vi "meTEC_Read_ID 101_Hardware Version.vi"(8 "error in (no error)":errorcluster, 9 "TEC Configuration_IN":T1={"VISA resource name"="", "Device Address"=2}, 10 "Sequence No.":u32=5552) -> (0 "error out":errorcluster, 1 "TEC Configuration_OUT":T1={"VISA resource name"="", "Device Address"=2}, 2 "Hardware Version (ID 101) [I32]":i32, 3 "Hardware Version (ID 101) [String]":string)   [LabVIEW 2023]
uses:
  TypeDefs/meTEC_Configuration.ctl
panel:
  # "--- Inputs ---"
  # "--- Outputs ---"
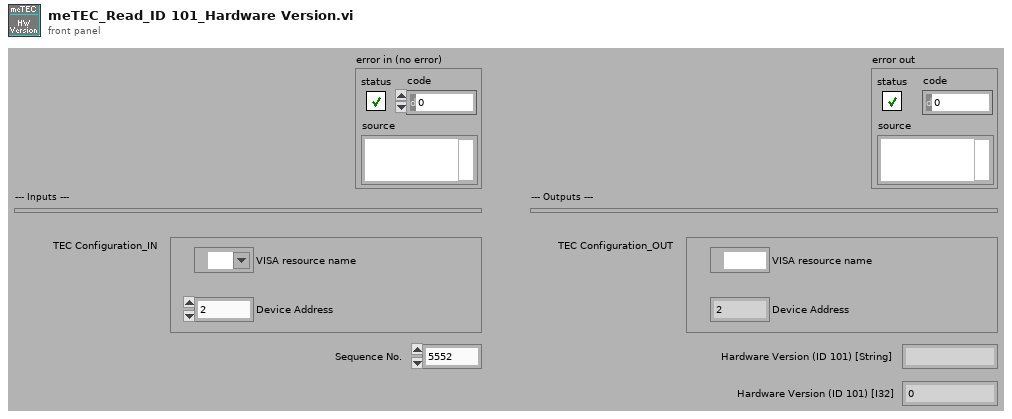
[diagram p1: front panel]
types:
  T1 = typedef "meTEC_Configuration.ctl" = cluster{"VISA resource name":refnum<visa-resource-name>, "Device Address":u16}
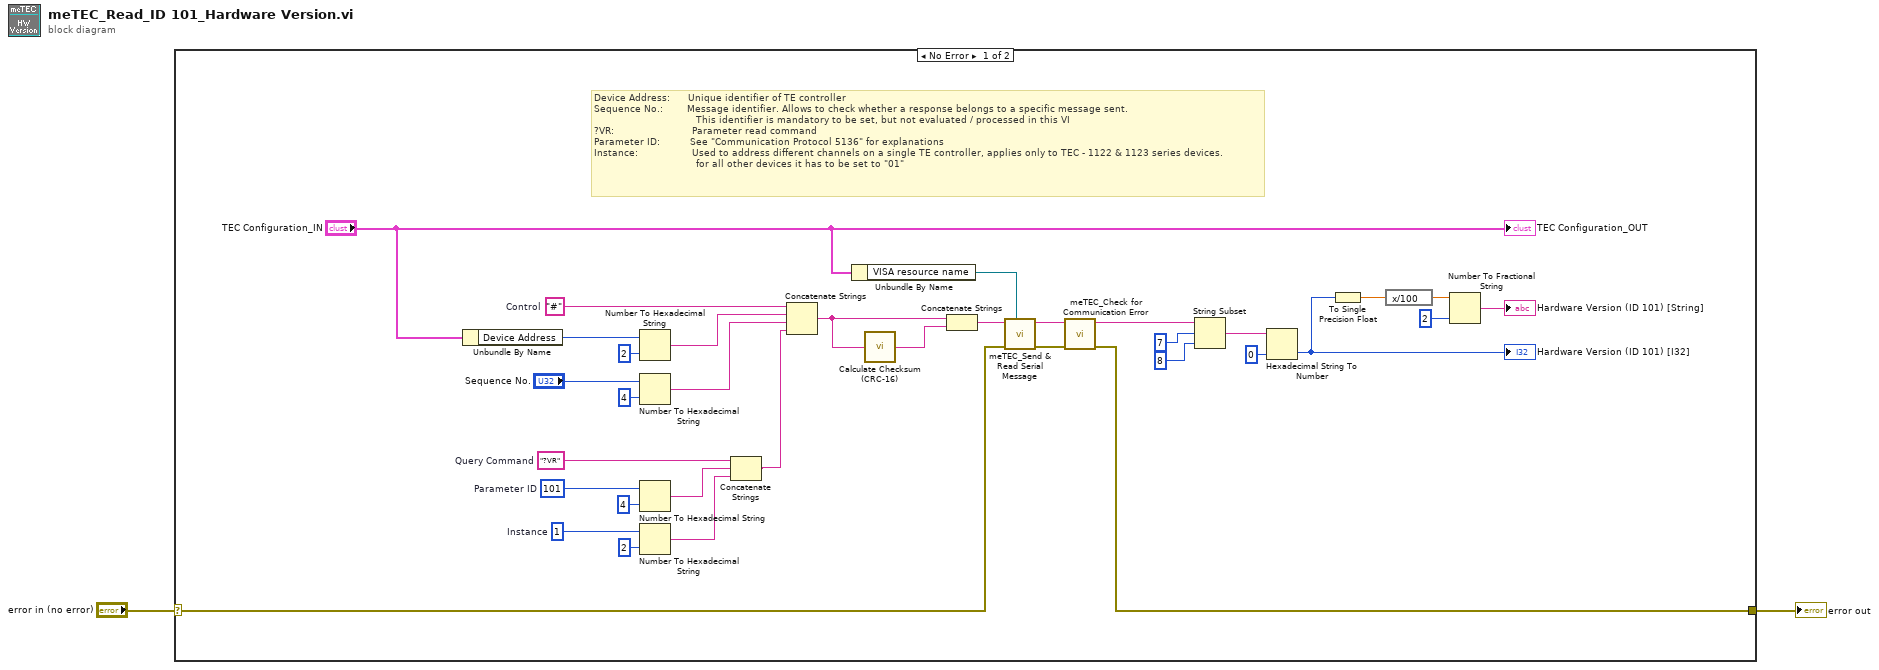
[diagram p0: block diagram]
diagram:
  n1 = case shown="No Error" "error in (no error)" {
    selector: "error in (no error)" -> [w20 w37]
    tunnel: [w5 w37] -> w2
    frame No Error {
      w6 = u8 1  # Instance
      w25 = 101  # Parameter ID
      w26 = "?VR"  # Query Command
      w34 = "#"  # Control
      # "Device Address:      Unique identifier of TE controller\nSequence No.:        Message identifier. Allows to check whether a response belongs to a specific message sent.\n                                  This identifier is mandatory to be set, but not evaluated / processed in this VI\n?VR:                          Parameter read command\nParameter ID:          See \"Communication Protocol 5136\" for explanations\nInstance:                  Used to address different channels on a single TE controller, applies only to TEC - 1122 & 1123 series devices.\n                                  for all other devices it has to be set to \"01\""
      n2 = Unbundle By Name("TEC Configuration_IN") -> ("Device Address"=w12:u16)
      n3 = Number To Hexadecimal String(1:i16 2 ("width (-)"), 2:w12) -> (0:w29:string)
      n4 = Number To Hexadecimal String(1:i16 4 ("width (-)"), 2:"Sequence No.") -> (0:w33:string)
      n5 = Number To Hexadecimal String(1:i16 4 ("width (-)"), 2:w25) -> (0:w27:string)
      n6 = Number To Hexadecimal String(1:i16 2 ("width (-)"), 2:w6) -> (0:w17:string)
      n7 = Concatenate Strings(w26, w27, w17) -> (w23:string)
      n8 = Concatenate Strings(w34, w29, w33, w23) -> (w32:string)
      n9 = Unbundle By Name("TEC Configuration_IN") -> ("VISA resource name"=w13:refnum<visa-resource-name>)
      n10 = call "Calculate Checksum (CRC-16).vi"("Message"=w32) -> ("CRC [String]"=w31:string)  [unwired: 1 in]
      n11 = Concatenate Strings(w32, w31) -> (w28:string)
      n12 = call "meTEC_Send & Read Serial Message.vi"("VISA resource name"=w13, "error in (no error)"=w20, "Serial Message"=w28) -> ("error out"=w19:errorcluster, "Serial Message_Read"=w4:string)  [unwired: 7 in]
      n13 = call "meTEC_Check for Communication Error.vi"("error in (no error)"=w19, "Serial Message_IN"=w4) -> ("error out"=w5:errorcluster, "Serial Message_OUT"=w3:string)  [unwired: 8 in]
      n14 = String Subset(string=w3, offset (0)=7, length (rest)=8 ("length (rest)")) -> (substring=w15:string)
      n15 = Hexadecimal String To Number(string=w15, default (0uL)=0 ("default (0 U32)")) -> (number=w14:i32)  [unwired: 1 in, 1 out]
      "Hardware Version (ID 101) [I32]" <- w14
      n16 = To Single Precision Float(number=w14) -> (single precision float=w8:sgl)
      n17 = expression code="x/100"(w8) -> (w9:sgl)
      n18 = Number To Fractional String(number=w9, precision (6)=i16 2) -> (F-format string=→"Hardware Version (ID 101) [String]":string)  [unwired: 2 in]
      "TEC Configuration_OUT" <- "TEC Configuration_IN"
    }
    frame Error {
    }
  }
  "error out" <- w2
